vi "SUPERVISORIO.vi"() -> ()   [LabVIEW 2018]
uses:
  <vilib>/Instr/_visa.llb/VISA Configure Serial Port (Instr).vi
panel:
  out "Aquec. Alta":bool
  out "Refrig. Alta":bool
  in  "Aquecedor 1":bool
  in  "Aquecedor 3":bool
  in  "Aquecedor 2":bool
  in  "Bomba Tanque":bool
  in  "Resist. Tanque":bool
  in  "Válvula Água":bool
  in  "Bomba Fancoil":bool
  in  "Vent. Fancoil":bool
  in  "Variac":bool
  in  "Vent. Aquecedor":bool
  out "Umidade %":u8(slide) scale=0.0..100.0
  out "Ambiente C°":dbl(slide) scale=0.0..100.0
  in  "Liga / Desl":bool
  out "Refrig. Baixa":bool
  in  "SetPoint":dbl
  out "Aquec. Baixa":bool
  out "Tanque":dbl(slide) scale=-50.0..150.0
  out "Retorno":dbl(slide) scale=-50.0..150.0
  out "Filtro de gás":dbl(slide) scale=-50.0..150.0
  out "Condensador":dbl(slide) scale=-50.0..150.0
  out "Ent. Água":dbl(slide) scale=-50.0..150.0
  out "Compressor":dbl(slide) scale=-50.0..150.0
  in  "stop":bool
  in  "Porta COM":refnum<visa-resource-name> caption="VISA resource name"
  # "Automação - Sala de Teste"
  # "Sensores de Temperatura - C°"
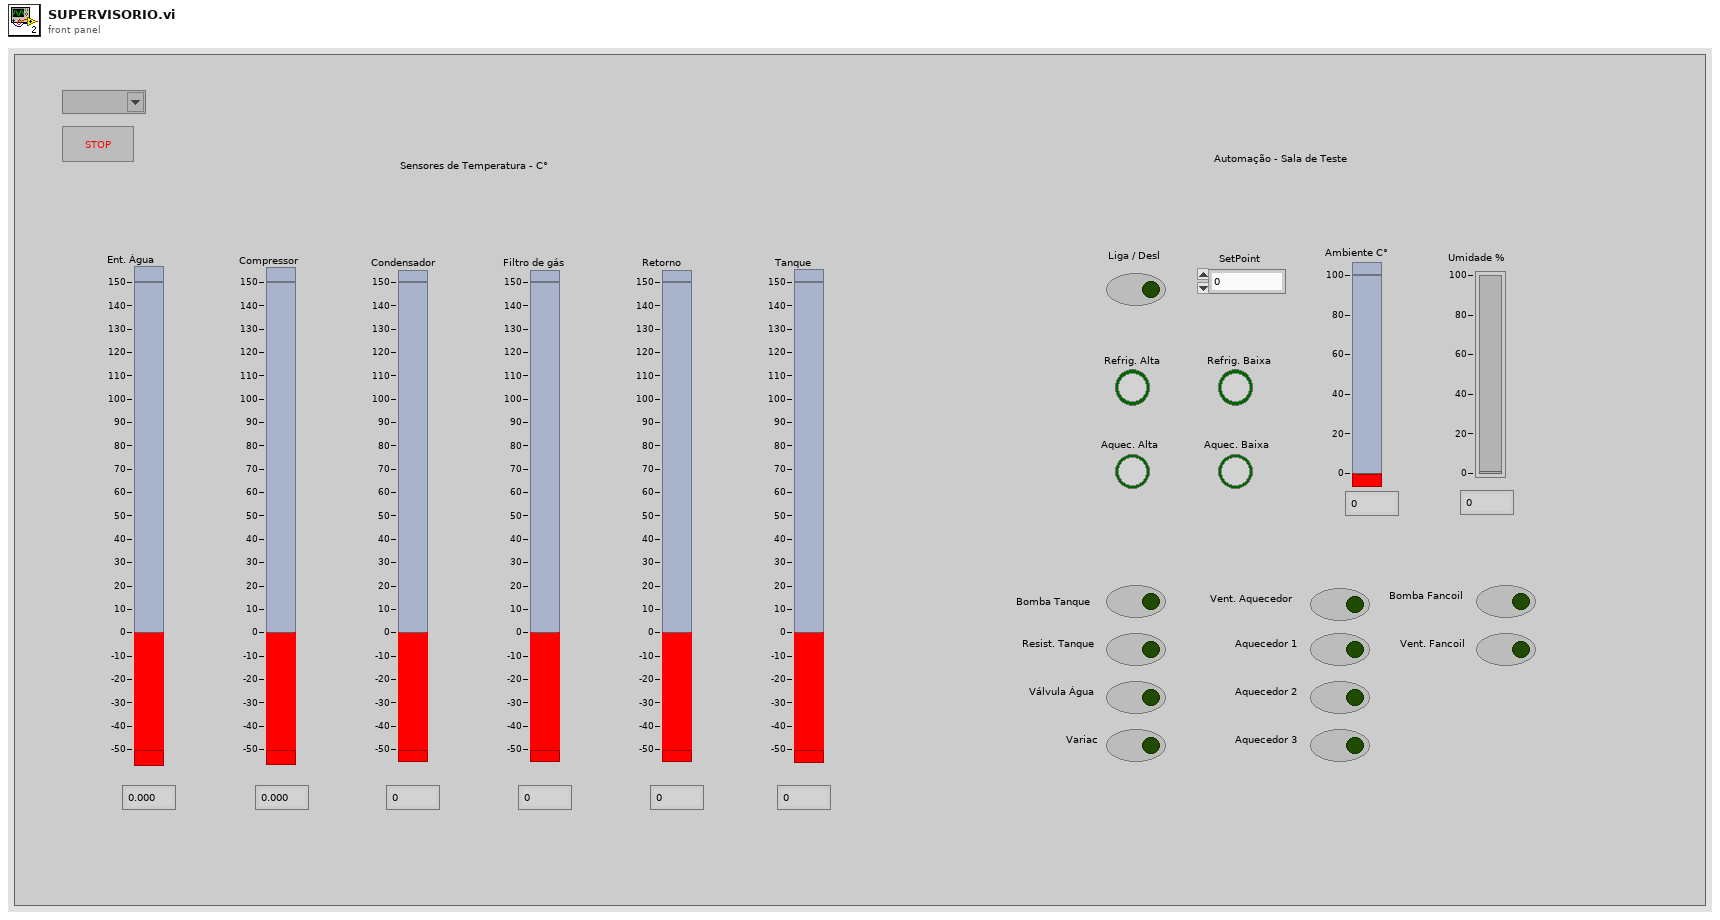
[diagram p1: front panel]
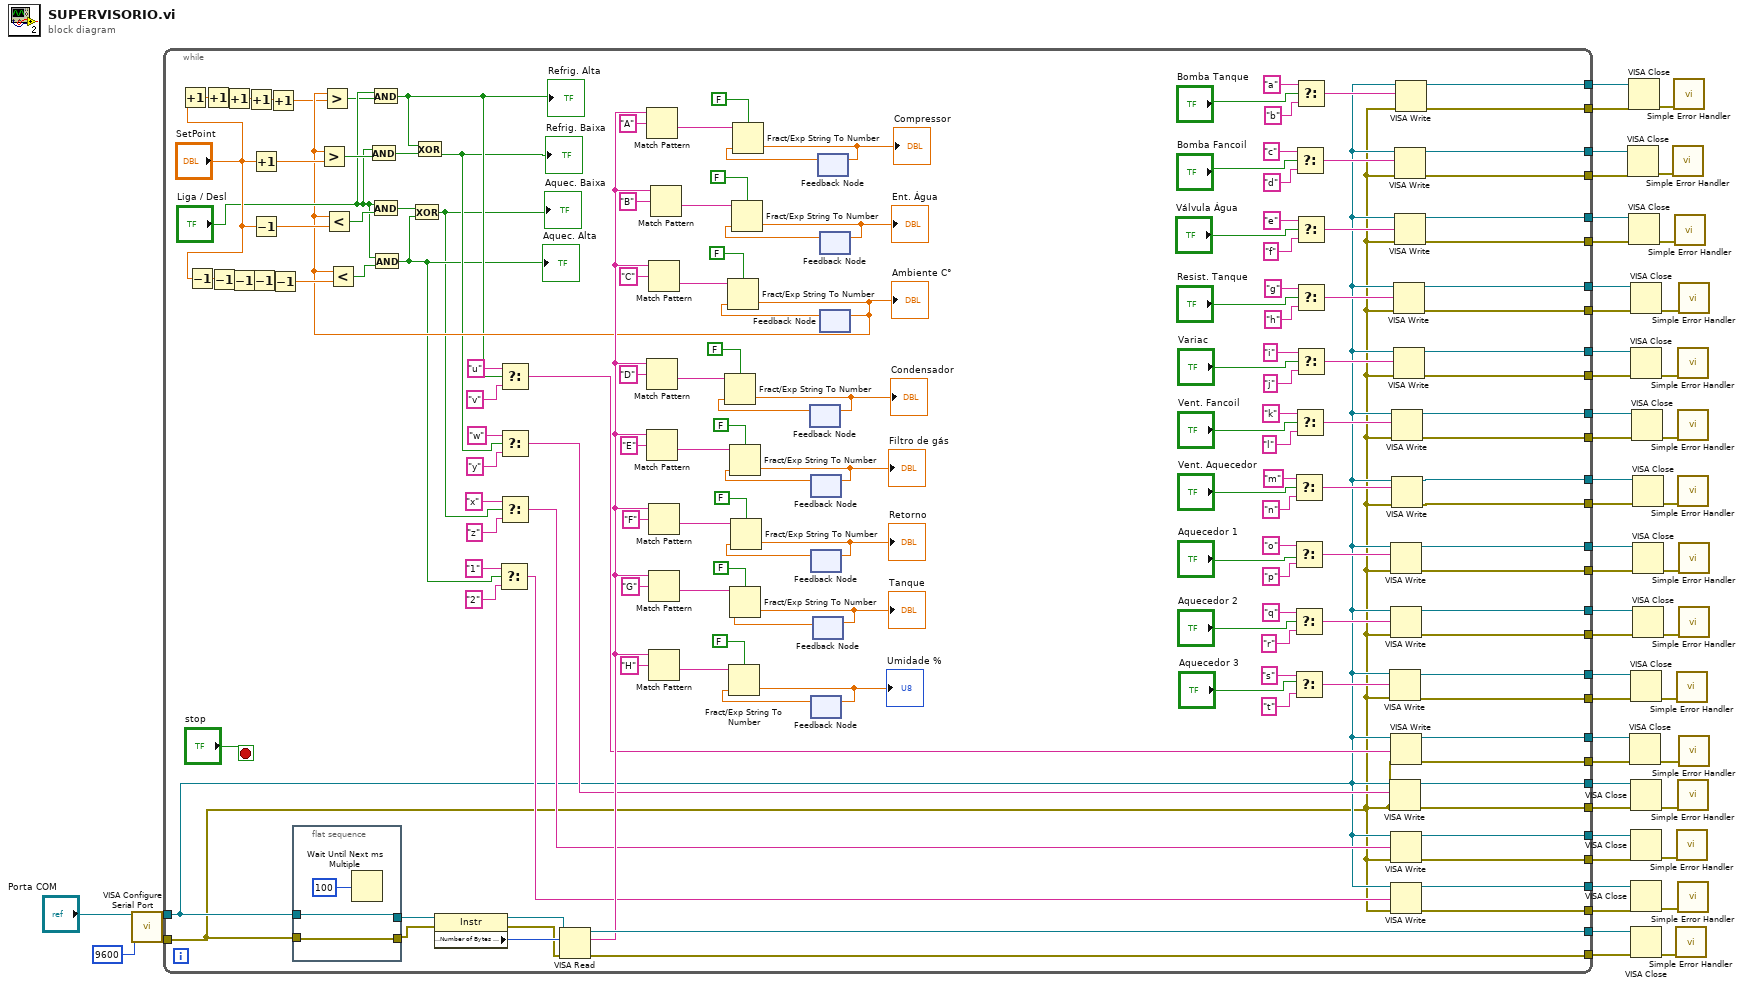
[diagram p0: block diagram]
diagram:
  n1 = call-poly "VISA Configure Serial Port"("VISA resource name"="Porta COM", "baud rate (9600)"=u32 9600) -> ("VISA resource name out"=w44:refnum<visa-resource-name>, "error out"=w43:errorcluster)  [unwired: 12 in]
  n2 = while {
    tunnel: w44 -> [w62]
    tunnel: w43 -> [w61]
    tunnel: [w193] -> w48
    tunnel: [w192] -> w47
    tunnel: [w155] -> w42
    tunnel: [w154] -> w41
    tunnel: [w153] -> w40
    tunnel: [w152] -> w39
    tunnel: [w151] -> w38
    tunnel: [w150] -> w37
    tunnel: [w149] -> w36
    tunnel: [w148] -> w35
    tunnel: [w147] -> w34
    tunnel: [w146] -> w33
    tunnel: [w145] -> w32
    tunnel: [w144] -> w31
    tunnel: [w143] -> w30
    tunnel: [w142] -> w29
    tunnel: [w141] -> w28
    tunnel: [w140] -> w27
    tunnel: [w139] -> w26
    tunnel: [w138] -> w25
    tunnel: [w137] -> w24
    tunnel: [w136] -> w23
    tunnel: [w74] -> w22
    tunnel: [w73] -> w21
    tunnel: [w70] -> w20
    tunnel: [w69] -> w19
    tunnel: [w68] -> w18
    tunnel: [w67] -> w17
    tunnel: [w66] -> w16
    tunnel: [w65] -> w15
    stop <- "stop" stop-if-true
    n3 = Increment(x="SetPoint") -> (x+1=w92:dbl)
    n4 = Decrement(x="SetPoint") -> (x-1=w88:dbl)
    n5 = Increment(x=w92) -> (x+1=w91:dbl)
    n6 = Decrement(x=w88) -> (x-1=w87:dbl)
    n7 = Increment(x=w91) -> (x+1=w90:dbl)
    n8 = Decrement(x=w87) -> (x-1=w86:dbl)
    n9 = Increment(x=w90) -> (x+1=w89:dbl)
    n10 = Decrement(x=w86) -> (x-1=w85:dbl)
    n11 = Increment(x="SetPoint") -> (x+1=w185:dbl)
    n12 = Decrement(x="SetPoint") -> (x-1=w186:dbl)
    n13 = Increment(x=w89) -> (x+1=w56:dbl)
    n14 = Decrement(x=w85) -> (x-1=w83:dbl)
    n15 = flat-sequence {
      tunnel: [w206] -> w64
      tunnel: [w205] -> w63
      tunnel: w62 -> [w206]
      tunnel: w61 -> [w205]
      frame #0 {
        n16 = Wait Until Next ms Multiple(millisecond multiple=u32 100 ("millisecond timer value")) -> ()  [unwired: 1 out]
      }
    }
    n17 = property class="Instr"(reference=w64, error in=w63) -> (reference out=w157:refnum<visa-resource-name>, error out=w156:errorcluster, "Serial Settings:Number of Bytes at Serial Port"=w204:u32)
    n18 = VISA Read(VISA resource name=w157, byte count=w204, error in (no error)=w156) -> (VISA resource name out=w193:refnum<visa-resource-name>, read buffer=w162:string, error out=w192:errorcluster)  [unwired: 1 out]
    n19 = Match Pattern(string=w162, regular expression="A") -> (after substring=w200:string)  [unwired: 1 in, 3 out]
    n20 = Match Pattern(string=w162, regular expression="D") -> (after substring=w175:string)  [unwired: 1 in, 3 out]
    n21 = Match Pattern(string=w162, regular expression="E") -> (after substring=w174:string)  [unwired: 1 in, 3 out]
    n22 = Match Pattern(string=w162, regular expression="C") -> (after substring=w190:string)  [unwired: 1 in, 3 out]
    n23 = Match Pattern(string=w162, regular expression="F") -> (after substring=w173:string)  [unwired: 1 in, 3 out]
    n24 = Match Pattern(string=w162, regular expression="G") -> (after substring=w172:string)  [unwired: 1 in, 3 out]
    n25 = Match Pattern(string=w162, regular expression="H") -> (after substring=w161:string)  [unwired: 1 in, 3 out]
    n26 = Match Pattern(string=w162, regular expression="B") -> (after substring=w199:string)  [unwired: 1 in, 3 out]
    n27 = feedback #1() -> (w171:dbl)  [unwired: 1 in]
    n28 = Fract/Exp String To Number(use system decimal point (T)=FALSE, string=w175, default (0 dbl)=w171) -> (number=w170:dbl)  [unwired: 1 in, 1 out]
    "Condensador" <- w170
    n29 = feedback-in #1(w170) -> ()
    n30 = feedback #2() -> (w169:dbl)  [unwired: 1 in]
    n31 = Fract/Exp String To Number(use system decimal point (T)=FALSE, string=w174, default (0 dbl)=w169) -> (number=w168:dbl)  [unwired: 1 in, 1 out]
    "Filtro de gás" <- w168
    n32 = feedback-in #2(w168) -> ()
    n33 = feedback #3() -> (w167:dbl)  [unwired: 1 in]
    n34 = Fract/Exp String To Number(use system decimal point (T)=FALSE, string=w173, default (0 dbl)=w167) -> (number=w166:dbl)  [unwired: 1 in, 1 out]
    "Retorno" <- w166
    n35 = feedback-in #3(w166) -> ()
    n36 = feedback #4() -> (w159:dbl)  [unwired: 1 in]
    n37 = Fract/Exp String To Number(use system decimal point (T)=FALSE, string=w161, default (0 dbl)=w159) -> (number=w158:dbl)  [unwired: 1 in, 1 out]
    "Umidade %" <- w158
    n38 = feedback-in #4(w158) -> ()
    n39 = feedback #5() -> (w165:dbl)  [unwired: 1 in]
    n40 = Fract/Exp String To Number(use system decimal point (T)=FALSE, string=w172, default (0 dbl)=w165) -> (number=w164:dbl)  [unwired: 1 in, 1 out]
    "Tanque" <- w164
    n41 = feedback-in #5(w164) -> ()
    n42 = feedback #6() -> (w196:dbl)  [unwired: 1 in]
    n43 = Fract/Exp String To Number(use system decimal point (T)=FALSE, string=w200, default (0 dbl)=w196) -> (number=w184:dbl)  [unwired: 1 in, 1 out]
    "Compressor" <- w184
    n44 = feedback-in #6(w184) -> ()
    n45 = feedback #7() -> (w194:dbl)  [unwired: 1 in]
    n46 = Fract/Exp String To Number(use system decimal point (T)=FALSE, string=w199, default (0 dbl)=w194) -> (number=w195:dbl)  [unwired: 1 in, 1 out]
    "Ent. Água" <- w195
    n47 = feedback-in #7(w195) -> ()
    n48 = feedback #8() -> (w188:dbl)  [unwired: 1 in]
    n49 = Fract/Exp String To Number(use system decimal point (T)=FALSE, string=w190, default (0 dbl)=w188) -> (number=w57:dbl)  [unwired: 1 in, 1 out]
    "Ambiente C°" <- w57
    n50 = Greater?(x=w57, y=w185) -> (0:w60:bool)
    n51 = Greater?(x=w57, y=w56) -> (0:w58:bool)
    n52 = Less?(x=w57, y=w186) -> (x < y?=w187:bool)
    n53 = Less?(x=w57, y=w83) -> (x < y?=w84:bool)
    n54 = And(x="Liga / Desl", y=w60) -> (x .and. y?=w54:bool)
    n55 = And(x="Liga / Desl", y=w58) -> (x .and. y?=w55:bool)
    "Refrig. Alta" <- w55
    n56 = And(x="Liga / Desl", y=w187) -> (x .and. y?=w52:bool)
    n57 = And(x="Liga / Desl", y=w84) -> (x .and. y?=w51:bool)
    "Aquec. Alta" <- w51
    n58 = Exclusive Or(1:w51, 2:w52) -> (0:w50:bool)
    "Aquec. Baixa" <- w50
    n59 = Exclusive Or(1:w54, 2:w55) -> (0:w53:bool)
    "Refrig. Baixa" <- w53
    n60 = Select(t="1", s=w51, f="2") -> (s? t:f=w71:string)
    n61 = Select(t="u", s=w55, f="v") -> (s? t:f=w93:string)
    n62 = Select(t="w", s=w53, f="y") -> (s? t:f=w75:string)
    n63 = Select(t="x", s=w50, f="z") -> (s? t:f=w72:string)
    n64 = feedback-in #8(w57) -> ()
    n65 = Select(t="m", s="Vent. Aquecedor", f="n") -> (s? t:f=w109:string)
    n66 = Select(t="o", s="Aquecedor 1", f="p") -> (s? t:f=w105:string)
    n67 = Select(t="q", s="Aquecedor 2", f="r") -> (s? t:f=w101:string)
    n68 = Select(t="s", s="Aquecedor 3", f="t") -> (s? t:f=w97:string)
    n69 = Select(t="c", s="Bomba Fancoil", f="d") -> (s? t:f=w129:string)
    n70 = Select(t="k", s="Vent. Fancoil", f="l") -> (s? t:f=w113:string)
    n71 = Select(t="a", s="Bomba Tanque", f="b") -> (s? t:f=w132:string)
    n72 = Select(t="e", s="Válvula Água", f="f") -> (s? t:f=w125:string)
    n73 = Select(t="g", s="Resist. Tanque", f="h") -> (s? t:f=w121:string)
    n74 = Select(t="i", s="Variac", f="j") -> (s? t:f=w117:string)
    n75 = VISA Write(VISA resource name=w62, write buffer=w97, error in (no error)=w61) -> (VISA resource name out=w137:refnum<visa-resource-name>, error out=w136:errorcluster)  [unwired: 1 out]
    n76 = VISA Write(VISA resource name=w62, write buffer=w75, error in (no error)=w61) -> (VISA resource name out=w70:refnum<visa-resource-name>, error out=w69:errorcluster)  [unwired: 1 out]
    n77 = VISA Write(VISA resource name=w62, write buffer=w105, error in (no error)=w61) -> (VISA resource name out=w141:refnum<visa-resource-name>, error out=w140:errorcluster)  [unwired: 1 out]
    n78 = VISA Write(VISA resource name=w62, write buffer=w101, error in (no error)=w61) -> (VISA resource name out=w139:refnum<visa-resource-name>, error out=w138:errorcluster)  [unwired: 1 out]
    n79 = VISA Write(VISA resource name=w62, write buffer=w93, error in (no error)=w61) -> (VISA resource name out=w74:refnum<visa-resource-name>, error out=w73:errorcluster)  [unwired: 1 out]
    n80 = VISA Write(VISA resource name=w62, write buffer=w72, error in (no error)=w61) -> (VISA resource name out=w68:refnum<visa-resource-name>, error out=w67:errorcluster)  [unwired: 1 out]
    n81 = VISA Write(VISA resource name=w62, write buffer=w71, error in (no error)=w61) -> (VISA resource name out=w66:refnum<visa-resource-name>, error out=w65:errorcluster)  [unwired: 1 out]
    n82 = VISA Write(VISA resource name=w62, write buffer=w113, error in (no error)=w61) -> (VISA resource name out=w145:refnum<visa-resource-name>, error out=w144:errorcluster)  [unwired: 1 out]
    n83 = VISA Write(VISA resource name=w62, write buffer=w109, error in (no error)=w61) -> (VISA resource name out=w143:refnum<visa-resource-name>, error out=w142:errorcluster)  [unwired: 1 out]
    n84 = VISA Write(VISA resource name=w62, write buffer=w121, error in (no error)=w61) -> (VISA resource name out=w149:refnum<visa-resource-name>, error out=w148:errorcluster)  [unwired: 1 out]
    n85 = VISA Write(VISA resource name=w62, write buffer=w117, error in (no error)=w61) -> (VISA resource name out=w147:refnum<visa-resource-name>, error out=w146:errorcluster)  [unwired: 1 out]
    n86 = VISA Write(VISA resource name=w62, write buffer=w129, error in (no error)=w61) -> (VISA resource name out=w153:refnum<visa-resource-name>, error out=w152:errorcluster)  [unwired: 1 out]
    n87 = VISA Write(VISA resource name=w62, write buffer=w125, error in (no error)=w61) -> (VISA resource name out=w151:refnum<visa-resource-name>, error out=w150:errorcluster)  [unwired: 1 out]
    n88 = VISA Write(VISA resource name=w62, write buffer=w132, error in (no error)=w61) -> (VISA resource name out=w155:refnum<visa-resource-name>, error out=w154:errorcluster)  [unwired: 1 out]
  }
  n89 = VISA Close(VISA resource name=w40, error in (no error)=w39) -> (error out=w13:errorcluster)
  n90 = VISA Close(VISA resource name=w42, error in (no error)=w41) -> (error out=w14:errorcluster)
  n91 = VISA Close(VISA resource name=w38, error in (no error)=w37) -> (error out=w12:errorcluster)
  n92 = VISA Close(VISA resource name=w22, error in (no error)=w21) -> (error out=w4:errorcluster)
  n93 = VISA Close(VISA resource name=w36, error in (no error)=w35) -> (error out=w11:errorcluster)
  n94 = VISA Close(VISA resource name=w34, error in (no error)=w33) -> (error out=w10:errorcluster)
  n95 = VISA Close(VISA resource name=w24, error in (no error)=w23) -> (error out=w5:errorcluster)
  n96 = VISA Close(VISA resource name=w20, error in (no error)=w19) -> (error out=w3:errorcluster)
  n97 = VISA Close(VISA resource name=w18, error in (no error)=w17) -> (error out=w2:errorcluster)
  n98 = VISA Close(VISA resource name=w16, error in (no error)=w15) -> (error out=w1:errorcluster)
  n99 = VISA Close(VISA resource name=w48, error in (no error)=w47) -> (error out=w46:errorcluster)
  n100 = VISA Close(VISA resource name=w32, error in (no error)=w31) -> (error out=w9:errorcluster)
  n101 = VISA Close(VISA resource name=w30, error in (no error)=w29) -> (error out=w8:errorcluster)
  n102 = VISA Close(VISA resource name=w28, error in (no error)=w27) -> (error out=w7:errorcluster)
  n103 = VISA Close(VISA resource name=w26, error in (no error)=w25) -> (error out=w6:errorcluster)
  n104 = call <vilib>:"Simple Error Handler.vi"("error in (no error)"=w13) -> ()  [unwired: 4 in, 5 out]
  n105 = call <vilib>:"Simple Error Handler.vi"("error in (no error)"=w14) -> ()  [unwired: 4 in, 5 out]
  n106 = call <vilib>:"Simple Error Handler.vi"("error in (no error)"=w12) -> ()  [unwired: 4 in, 5 out]
  n107 = call <vilib>:"Simple Error Handler.vi"("error in (no error)"=w46) -> ()  [unwired: 4 in, 5 out]
  n108 = call <vilib>:"Simple Error Handler.vi"("error in (no error)"=w5) -> ()  [unwired: 4 in, 5 out]
  n109 = call <vilib>:"Simple Error Handler.vi"("error in (no error)"=w2) -> ()  [unwired: 4 in, 5 out]
  n110 = call <vilib>:"Simple Error Handler.vi"("error in (no error)"=w10) -> ()  [unwired: 4 in, 5 out]
  n111 = call <vilib>:"Simple Error Handler.vi"("error in (no error)"=w9) -> ()  [unwired: 4 in, 5 out]
  n112 = call <vilib>:"Simple Error Handler.vi"("error in (no error)"=w8) -> ()  [unwired: 4 in, 5 out]
  n113 = call <vilib>:"Simple Error Handler.vi"("error in (no error)"=w3) -> ()  [unwired: 4 in, 5 out]
  n114 = call <vilib>:"Simple Error Handler.vi"("error in (no error)"=w1) -> ()  [unwired: 4 in, 5 out]
  n115 = call <vilib>:"Simple Error Handler.vi"("error in (no error)"=w11) -> ()  [unwired: 4 in, 5 out]
  n116 = call <vilib>:"Simple Error Handler.vi"("error in (no error)"=w7) -> ()  [unwired: 4 in, 5 out]
  n117 = call <vilib>:"Simple Error Handler.vi"("error in (no error)"=w6) -> ()  [unwired: 4 in, 5 out]
  n118 = call <vilib>:"Simple Error Handler.vi"("error in (no error)"=w4) -> ()  [unwired: 4 in, 5 out]
